vi "main(Test DQMH modules).bak.vi"() -> ()   [LabVIEW 2018, in "Application.lvlib"]
uses:
  eMIC response.ctl
  DRV stand.ctl
  type defs/HW config.ctl
  eMICs Cluster.ctl
  SubVIs/App state data.ctl
  SubVIs/Trigger cluster.ctl
  type defs/DMM all config cluster.ctl
  type defs/DMM config cluster.ctl
  SubVIs/FGV DRV data.ctl
  SubVIs/DUT data Mode.ctl
  Instrument Drivers/LV_driver_MBrelay/type defs/FGV enum.ctl
  SubVIs/Step data.ctl
  DRV cluster 2.ctl
  <vilib>/ErrorRing/Error Ring.xnode
  Application.lvlib
  Switches Module/MB switches Module.lvlib
  MB 01 switches Module/MB 01 switches Module.lvlib
  DMM Module/DMM Module.lvlib
  v2_CE14/CE14_v2.lvlib
  Instrument Drivers/LV_driver_MBrelay/MB Relay.lvlib
panel:
  in  "milliseconds to wait":u32=1500
  in  "Log report":bool
  in  "10-1 delay":u32=70
  in  "6_1 delay2":u32=70
  in  "DMM delay":u32=10
  in  "6_1 delay":u32=150
  in  "1-10delay":u32=70
  in  "eMIC delay":u32=70
  in  "DRV number":u8=1 max=60
  in  "Test Single DRV":bool
  in  "Enum":T1(ring)=enum."Fixxed"
  out "Name":string
  out "SAP ID":string
  out "Progress":string
  out "DRV stand":T2
  in  "Auto/Man":bool
  out "DC Measure Completed":bool caption="DC Completed"
  in  "Test Channel 10":bool
  in  "Test Channel 9":bool
  in  "Test Channel 8":bool
  in  "Test Channel 7":bool
  in  "Test Channel 6":bool
  in  "Test Channel 5":bool
  in  "Test Channel 4":bool
  in  "Test Channel 3":bool
  in  "Test Channel 2":bool
  in  "Test Channel 1":bool
  in  "Shorted Circuits Test":bool
  out "CE14  Module did it":bool[](array[boolean])
  out "time elased(ms)":u32
  out "Inst. 9":bool
  in  "Exit":bool
  out "Inst. 8":bool
  out "Inst. 7":bool
  out "Inst. 6":bool
  out "Inst. 5":bool
  out "Inst. 4":bool
  out "Inst. 3":bool
  out "Inst. 2":bool
  out "Inst. 1":bool
  out "new Trigger?":bool
  out "last Trigger?":bool
  out "error out":errorcluster
  out "State log":string
  out "AC  Completed":bool caption="AC Completed"
  in  "Select CE14 eMIC Module Instance":i32(ring)=-1 items=["All"=-1, "1"=1, "2"=2, "3"=3, "4"=4, "5"=5, "6"=6]
  out "New board?":bool
  in  "Test":bool caption="Again"
  out "DRV 61":u32(colorbox)
  in  "Settings":bool
  in  "VIEW":bool caption="Again"
  out "DRV 60":u32(colorbox) caption="60"
  out "DRV 59":u32(colorbox) caption="59"
  out "DRV 58":u32(colorbox) caption="58"
  out "DRV 57":u32(colorbox) caption="57"
  out "DRV 56":u32(colorbox) caption="56"
  out "DRV 55":u32(colorbox) caption="55"
  out "DRV 54":u32(colorbox) caption="54"
  out "DRV 53":u32(colorbox) caption="53"
  out "DRV 52":u32(colorbox) caption="52"
  out "DRV 51":u32(colorbox) caption="51"
  out "DRV 50":u32(colorbox) caption="50"
  out "DRV 49":u32(colorbox) caption="49"
  out "DRV 48":u32(colorbox) caption="48"
  out "DRV 47":u32(colorbox) caption="47"
  out "DRV 46":u32(colorbox) caption="46"
  out "DRV 45":u32(colorbox) caption="45"
  out "DRV 44":u32(colorbox) caption="44"
  out "DRV 43":u32(colorbox) caption="43"
  out "DRV 42":u32(colorbox) caption="42"
  out "DRV 41":u32(colorbox) caption="41"
  out "DRV 40":u32(colorbox) caption="40"
  out "DRV 39":u32(colorbox) caption="39"
  out "DRV 38":u32(colorbox) caption="38"
  out "DRV 37":u32(colorbox) caption="37"
  out "DRV 36":u32(colorbox) caption="36"
  out "DRV 35":u32(colorbox) caption="35"
  out "DRV 34":u32(colorbox) caption="34"
  out "DRV 33":u32(colorbox) caption="33"
  out "DRV 32":u32(colorbox) caption="32"
  out "DRV 31":u32(colorbox) caption="31"
  out "DRV 30":u32(colorbox) caption="30"
  out "DRV 29":u32(colorbox) caption="29"
  out "DRV 28":u32(colorbox) caption="28"
  out "DRV 27":u32(colorbox) caption="27"
  out "DRV 26":u32(colorbox) caption="26"
  out "DRV 25":u32(colorbox) caption="25"
  out "DRV 24":u32(colorbox) caption="24"
  out "DRV 23":u32(colorbox) caption="23"
  out "DRV 22":u32(colorbox) caption="22"
  out "DRV 21":u32(colorbox) caption="21"
  out "DRV 20":u32(colorbox) caption="20"
  out "DRV 19":u32(colorbox) caption="19"
  out "DRV 18":u32(colorbox) caption="18"
  out "DRV 17":u32(colorbox) caption="17"
  out "DRV 16":u32(colorbox) caption="16"
  out "DRV 15":u32(colorbox) caption="15"
  out "DRV 14":u32(colorbox) caption="14"
  out "DRV 13":u32(colorbox) caption="13"
  out "DRV 12":u32(colorbox) caption="12"
  out "DRV 11":u32(colorbox) caption="11"
  out "DRV 10":u32(colorbox) caption="10"
  out "DRV 9":u32(colorbox) caption="9"
  out "DRV 8":u32(colorbox) caption="8"
  out "DRV 7":u32(colorbox) caption="7"
  out "DRV 6":u32(colorbox) caption="6"
  out "DRV 5":u32(colorbox) caption="5"
  out "DRV 4":u32(colorbox) caption="4"
  out "DRV 3":u32(colorbox) caption="3"
  out "DRV 2":u32(colorbox) caption="2"
  out "DRV 1":u32(colorbox) caption="1"
  out "version":string caption="Version"
  out "Module ID":i32
  in  "Tab Control":T3(tab)
  out "Short DRV":bool[][](array[boolean])
  in  "Mux 10-1":bool
  in  "mux 6-1":bool
  in  "Read Optos":bool
  in  "Select DMM's Current Input":bool
  in  "mux2-1(DMM I) encode":enum16{"DMM I (0.5)", "DMM I (12)"}(ring)
  in  "mux 6-1 data":T4(ring)
  in  "mux 10-1 data":T5(ring)
  in  "set value":bool
  in  "Set trigger value":bool
  out "trigger Value":bool
  in  "Read trigger":bool
  in  "Reset JIG":bool
  in  "eMIC":bool
  in  "DEMUX 1-10":bool
  in  "TurnON/OFF +5V":bool
  in  "5V Value":bool
  in  "demux1_10(x6)_encode":T6(ring)
  in  "eMIC 6 values":bool[](array[boolean])=[FALSE, FALSE, FALSE, FALSE, FALSE, FALSE]
  in  "DMM query":bool
  in  "connect DMM":bool
  in  "DMM read dual value":bool
  in  "config DMM":bool
  in  "Detector Rate":u8(ring)=2 items=["SLOW", "MID", "FAST"]
  in  "DCI range":dbl=0.5
  in  "DCV range":dbl=1000.0
  out "DCV(Volts)":dbl
  out "DCI(mA)":dbl
  out "DMM func?":string
  out "DMM range?":string
  in  "request AC-all":bool
  in  "Open COM eMIC":bool
  in  "check connected":bool
  out "eMIC 1":T7
  out "eMIC 2":T7
  out "eMIC 3":T7
  out "eMIC 4":T7
  out "eMIC 5":T7
  out "eMIC 6":T7
  out "EMIC connected":bool[](array[boolean])
  out "AC switches Module":bool
  out "DC Measure Module":bool
  out "DC Switches Module":bool
  out "AC Measure Module":bool
  # "HV-60D: ON-LINE TESTER FOR LED POWER DRIVER"
  # "60"
  # "6"
  # "12"
  # "18"
  # "24"
  # "30"
  # "36"
  # "42"
  # "48"
  # "54"
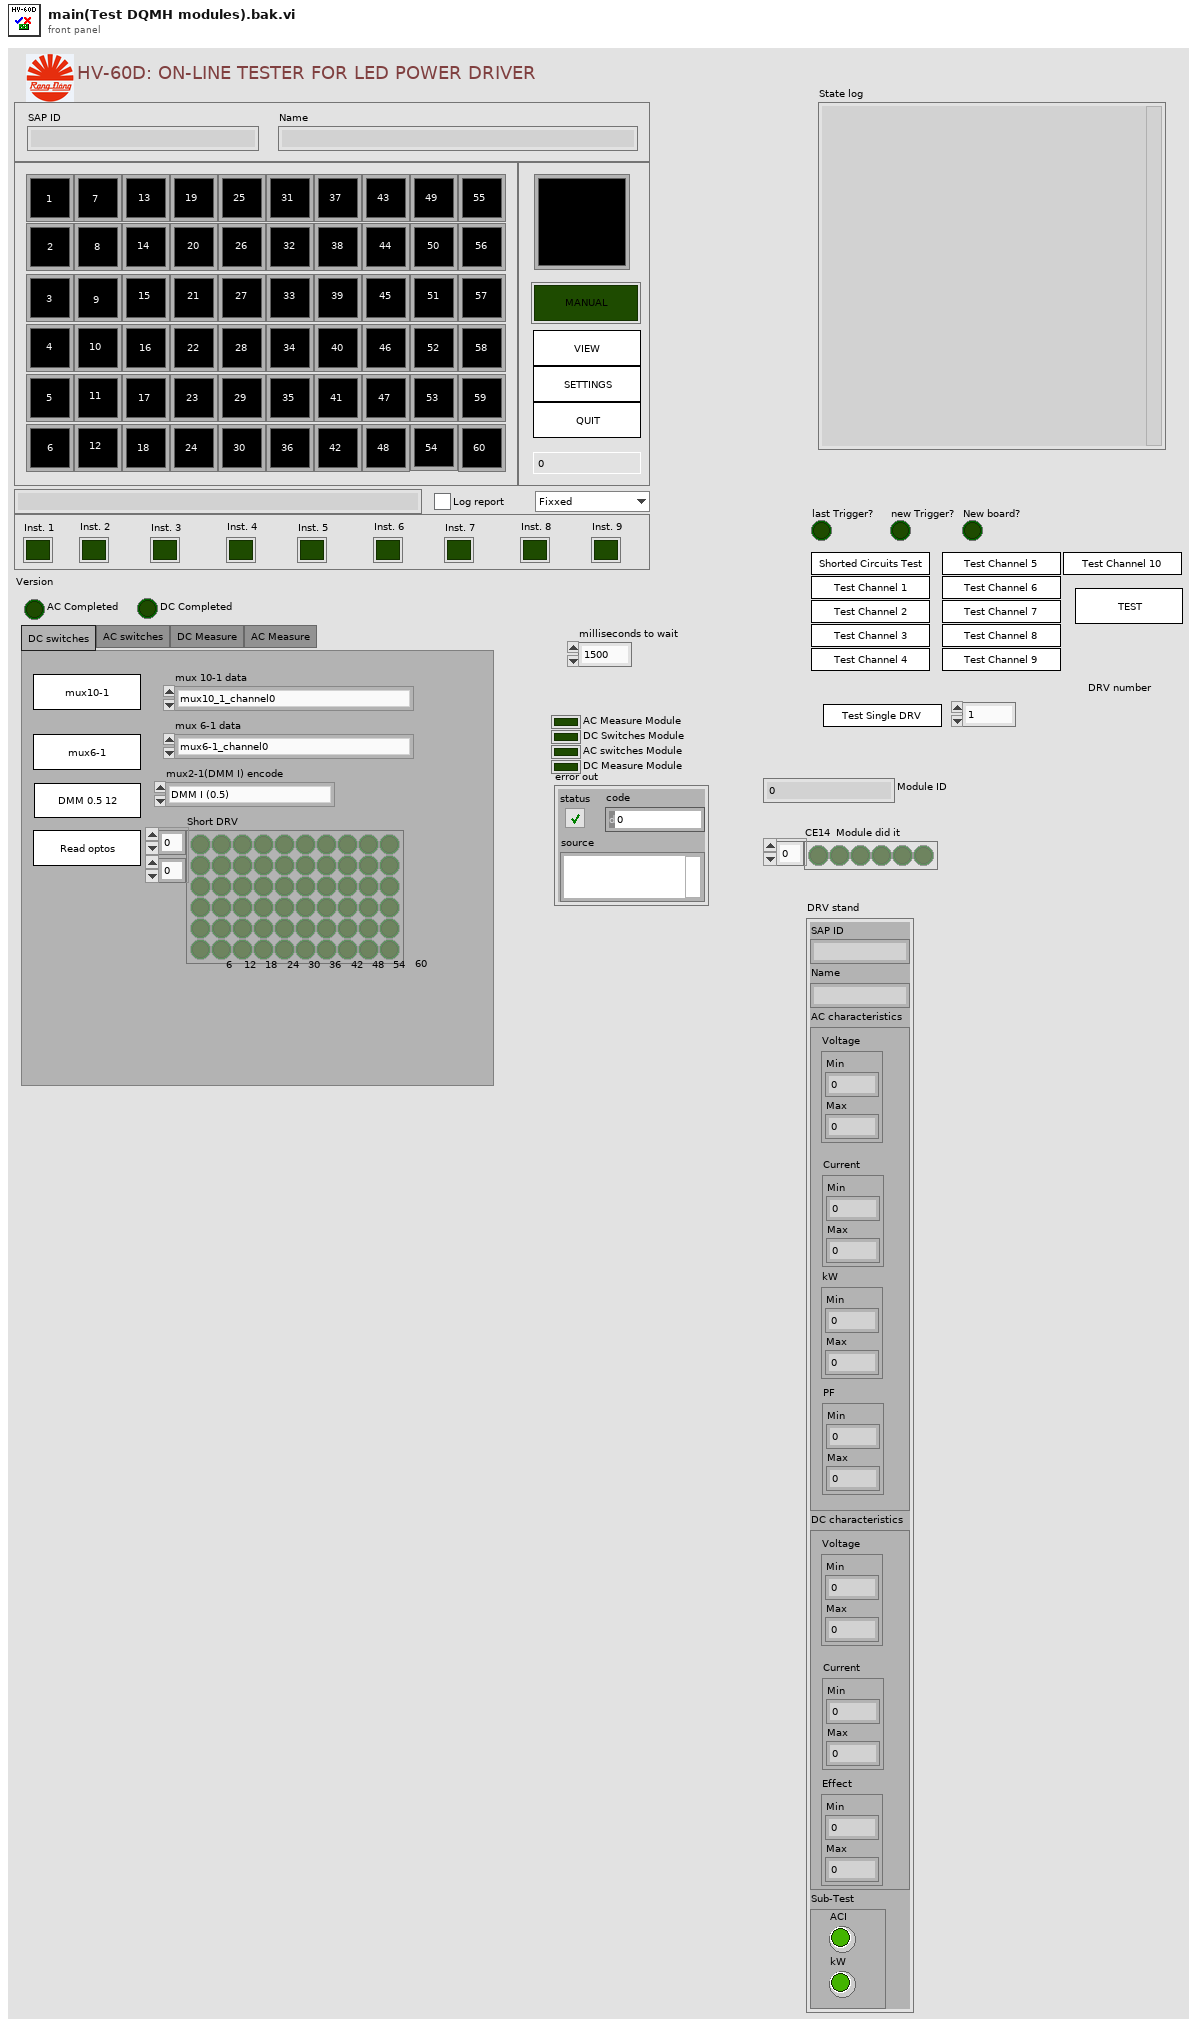
[diagram p1: front panel]
types:
  T1 = enum16{"All DRV", "Fixxed", "Pinpoint_JIG", "00037845(M26)"}
  T2 = typedef "Application.lvlib/DRV stand.ctl" = cluster{"SAP ID":string, "Name":string, "AC characteristics":cluster{"Voltage":cluster{"Min":dbl, "Max":dbl}, "Current":cluster{"Min":dbl, "Max":dbl}, "kW":cluster{"Min":dbl, "Max":dbl}, "PF":cluster{"Min":dbl, "Max":dbl}}, "DC characteristics":cluster{"Voltage":cluster{"Min":dbl, "Max":dbl}, "Current":cluster{"Min":dbl, "Max":dbl}, "Effect":cluster{"Min":dbl, "Max":dbl}}, "Sub-Test":cluster{"ACV":bool, "ACI":bool, "kW":bool, "PF":bool, "DCV":bool, "DCI":bool, "efficiency":bool}}
  T3 = enum32{"DC switches", "AC switches", "DC Measure", "AC Measure"}
  T4 = enum16{"mux6-1_channel0", "mux6_1_channel1_0", "mux6_1_channel1_1", "mux6-1_channel1_2", "mux6_1_channel1_3", "mux6_1_channel2_0", "mux6_1_channel2_1", "mux6_1_channel2_2", "mux6_1_channel2_3", "mux6_1_channel3_0", "mux6_1_channel3_1", "mux6_1_channel3_2", "mux6_1_channel3_3", "mux6_1_channel4_0", "mux6_1_channel4_1", "mux6_1_channel4_2", "mux6_1_channel4_3", "mux6_1_channel5_0", "mux6_1_channel5_1", "mux6_1_channel5_2", "mux6_1_channel5_3", "mux6_1_channel6_0", "mux6_1_channel6_1", "mux6_1_channel6_2", "mux6_1_channel6_3"}
  T5 = enum16{"mux10_1_channel0", "mux10_1_channel1", "mux10_1_channel2", "mux10_1_channel3", "mux10_1_channel4", "mux10_1_channel5", "mux10_1_channel6", "mux10_1_channel7", "mux10_1_channel8", "mux10_1_channel9", "mux10_1_channel10"}
  T6 = enum16{"demux1_10_channel0", "demux1_10_channel1", "demux1_10_channel2", "demux1_10_channel3", "demux1_10_channel4", "demux1_10_channel5", "demux1_10_channel6", "demux1_10_channel7", "demux1_10_channel8", "demux1_10_channel9", "demux1_10_channel10"}
  T7 = typedef "Application.lvlib/eMIC response.ctl" = cluster{"ACV":dbl, "ACI":dbl, "pF":dbl, "kW":dbl, "Freq":dbl, "kvar":dbl}
  T8 = typedef "Application.lvlib/eMICs Cluster.ctl" = cluster{"eMIC 1":T7, "eMIC 2":T7, "eMIC 3":T7, "eMIC 4":T7, "eMIC 5":T7, "eMIC 6":T7}
  T9 = typedef "Application.lvlib/HW config.ctl" = cluster{"DMM":string, "mux":string, "demux":string, "eMIC1":string, "eMIC2":string, "eMIC3":string, "eMIC4":string, "eMIC5":string, "eMIC6":string}
  T10 = typedef "Application.lvlib/Trigger cluster.ctl" = cluster{"new board?":bool, "new trigger":bool, "last trigger":bool}
  T11 = typedef "Application.lvlib/App state data.ctl" = cluster{"command":string, "command data":variant}
  T12 = typedef "CE14_v2.lvlib/Broadcast Events--cluster.ctl" = cluster{"Module Did Init":refnum<user-event>, "Status Updated":refnum<user-event>, "Error Reported":refnum<user-event>, "Module Did Stop":refnum<user-event>, "Update Module Execution Status":refnum<user-event>, "CE14 response data":refnum<user-event>}
  T13 = typedef "MB switches Module.lvlib/Broadcast Events--cluster.ctl" = cluster{"Module Did Init":refnum<user-event>, "Status Updated":refnum<user-event>, "Error Reported":refnum<user-event>, "Module Did Stop":refnum<user-event>, "Update Module Execution Status":refnum<user-event>}
  T14 = typedef "MB 01 switches Module.lvlib/Broadcast Events--cluster.ctl" = cluster{"Module Did Init":refnum<user-event>, "Status Updated":refnum<user-event>, "Error Reported":refnum<user-event>, "Module Did Stop":refnum<user-event>, "Update Module Execution Status":refnum<user-event>}
  T15 = typedef "DMM Module.lvlib/Broadcast Events--cluster.ctl" = cluster{"Module Did Init":refnum<user-event>, "Status Updated":refnum<user-event>, "Error Reported":refnum<user-event>, "Module Did Stop":refnum<user-event>, "Update Module Execution Status":refnum<user-event>}
  T16 = enum16{"open", "replace", "create", "open or create", "replace or create", "replace or create with confirmation"}
  T17 = typedef "Application.lvlib/DRV cluster 2.ctl" = cluster{"Shorted Circuit":bool, "AC voltage(volts)":dbl, "AC Current (mA)":dbl, "AC kW (W)":dbl, "AC pF ":dbl, "DC Voltage (Volts)":dbl, "DC Current (mA)":dbl, "DC kW (W)":dbl, "DRV Fail/Pass (T)":bool, "efficient (%)":dbl}
  T18 = enum32{"Invalid", "Standard", "Closed", "Hidden", "Minimized", "Maximized"}
  T19 = typedef "Application.lvlib/DMM all config cluster.ctl" = cluster{"DMM config cluster":T20, "mux2-1(DMM I) encode":enum16{"DMM I (0.5)", "DMM I (12)"}}
  T20 = typedef "Application.lvlib/DMM config cluster.ctl" = cluster{"DCV range":dbl, "DCI range":dbl, "Detector Rate":u8}
  T21 = typedef "Application.lvlib/DUT data Mode.ctl" = enum16{"range Limit", "Short Circuits", "AC parameter", "AC parameter 1", "DC parameter"}
  T22 = typedef "Application.lvlib/FGV DRV data.ctl" = enum16{"Init", "Write", "Read", "Process"}
  T23 = typedef "MB Relay.lvlib/FGV enum.ctl" = enum16{"Write", "Init FGV", "Read", "All OFF", "All ON"}
  T24 = typedef "CE14_eMIC.lvlib/CE14.data.ctl" = cluster{"string":string, "float":dbl, "Name":string}
  T25 = typedef "Application.lvlib/Step data.ctl" = cluster{"command":string, "Data":variant}
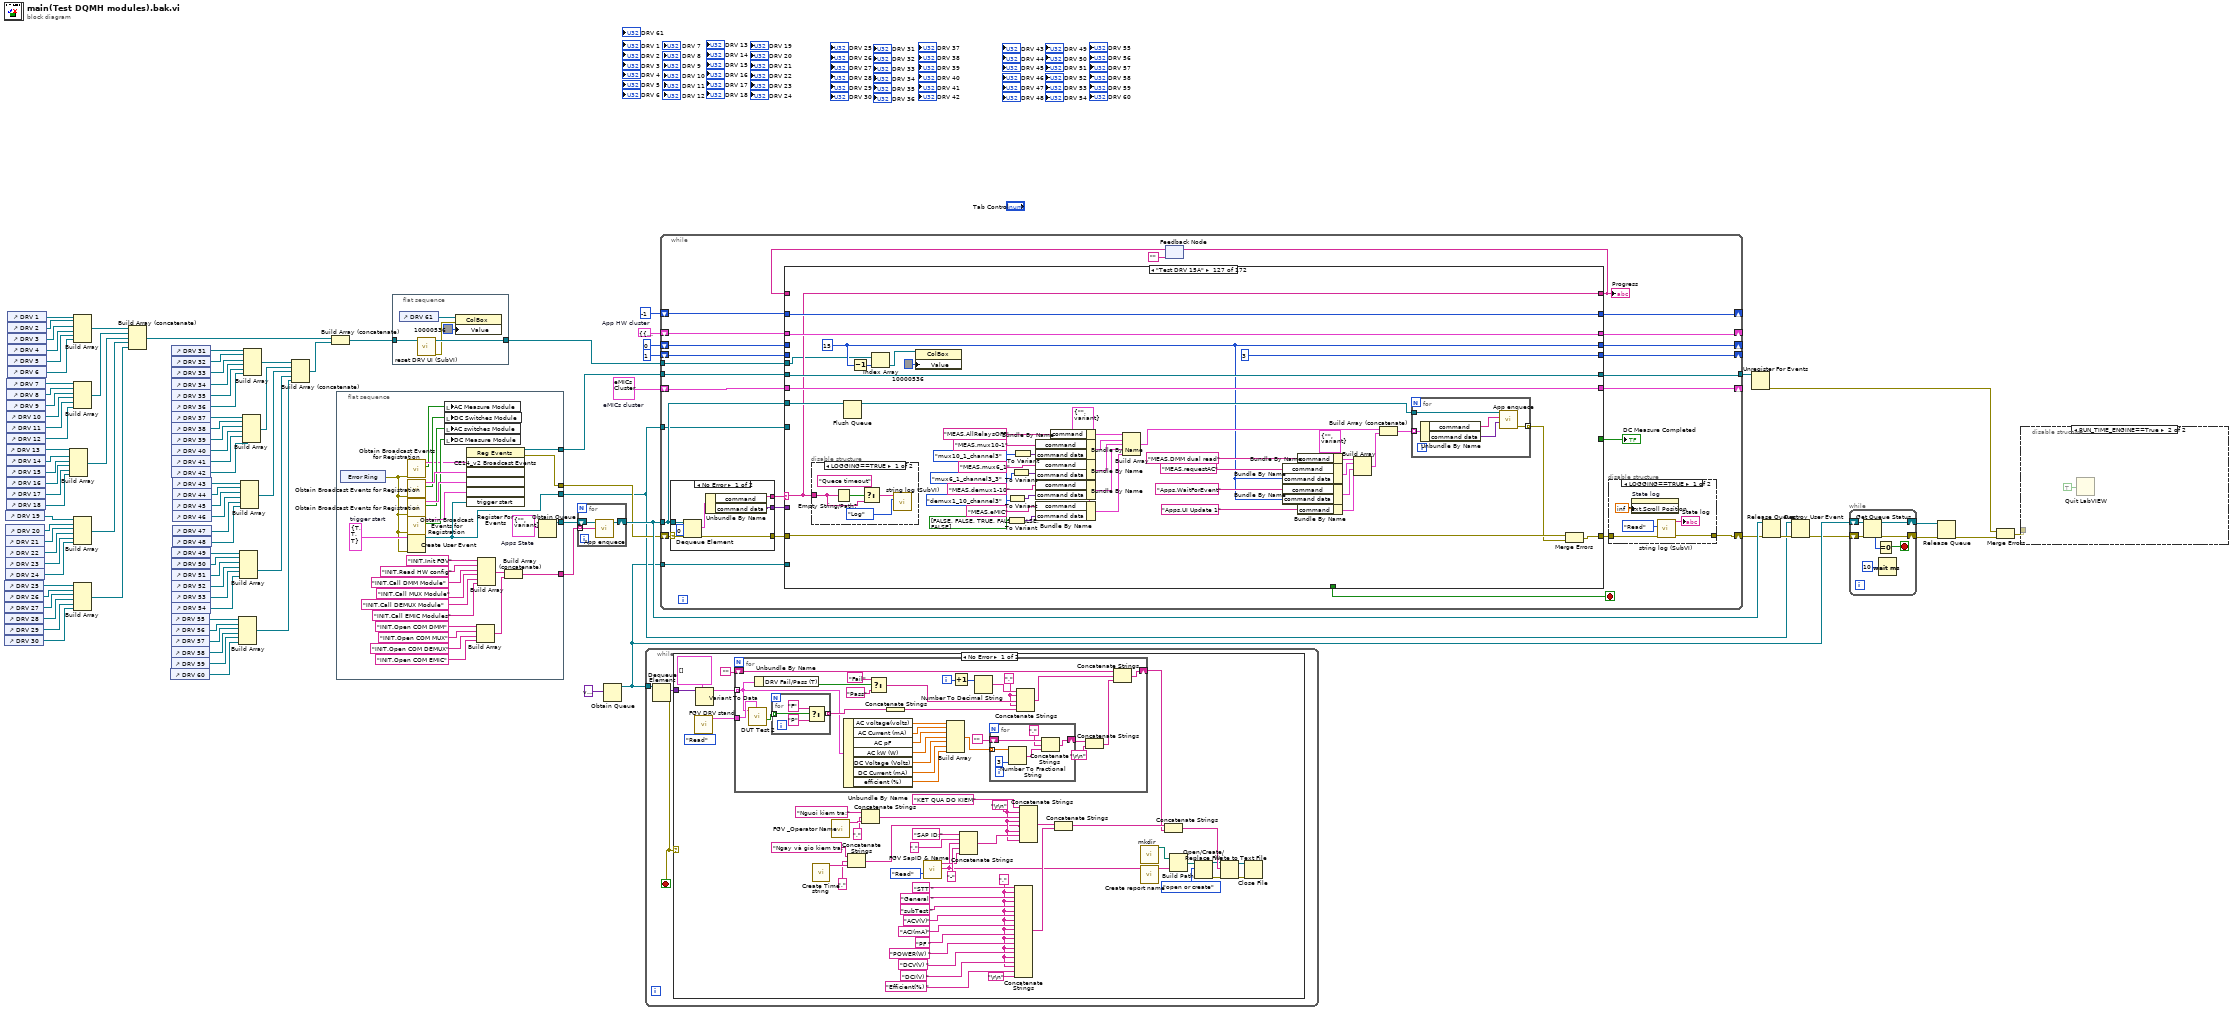
[diagram p0: block diagram]
diagram:
  w88 = T8 {"eMIC 1"={"ACV"=0.0, "ACI"=0.0, "pF"=0.0, "kW"=0.0, "Freq"=0.0, "kvar"=0.0}, "eMIC 2"={"ACV"=0.0, "ACI"=0.0, "pF"=0.0, "kW"=0.0, "Freq"=0.0, "kvar"=0.0}, "eMIC 3"={"ACV"=0.0, "ACI"=0.0, "pF"=0.0, "kW"=0.0, "Freq"=0.0, "kvar"=0.0}, "eMIC 4"={"ACV"=0.0, "ACI"=0.0, "pF"=0.0, "kW"=0.0, "Freq"=0.0, "kvar"=0.0}, "eMIC 5"={"ACV"=0.0, "ACI"=0.0, "pF"=0.0, "kW"=0.0, "Freq"=0.0, "kvar"=0.0}, "eMIC 6"={"ACV"=0.0, "ACI"=0.0, "pF"=0.0, "kW"=0.0, "Freq"=0.0, "kvar"=0.0}}  # eMICs cluster
  w93 = cluster{"HW config 2":T9} {"HW config 2"={"DMM"="COM15", "mux"="COM11", "demux"="COM16", "eMIC1"="COM13", "eMIC2"="COM6", "eMIC3"="COM9", "eMIC4"="COM10", "eMIC5"="COM12", "eMIC6"="COM11"}}  # App HW cluster
  n1 = control-ref of="DRV 25"() -> (w58:refnum<vi>)
  n2 = control-ref of="DRV 26"() -> (w59:refnum<vi>)
  n3 = control-ref of="DRV 27"() -> (w60:refnum<vi>)
  n4 = control-ref of="DRV 28"() -> (w61:refnum<vi>)
  n5 = control-ref of="DRV 29"() -> (w62:refnum<vi>)
  n6 = control-ref of="DRV 30"() -> (w63:refnum<vi>)
  n7 = control-ref of="DRV 21"() -> (w67:refnum<vi>)
  n8 = control-ref of="DRV 22"() -> (w66:refnum<vi>)
  n9 = control-ref of="DRV 23"() -> (w65:refnum<vi>)
  n10 = control-ref of="DRV 24"() -> (w64:refnum<vi>)
  n11 = control-ref of="DRV 19"() -> (w69:refnum<vi>)
  n12 = control-ref of="DRV 20"() -> (w68:refnum<vi>)
  n13 = control-ref of="DRV 13"() -> (w75:refnum<vi>)
  n14 = control-ref of="DRV 7"() -> (w81:refnum<vi>)
  n15 = control-ref of="DRV 8"() -> (w80:refnum<vi>)
  n16 = control-ref of="DRV 9"() -> (w79:refnum<vi>)
  n17 = control-ref of="DRV 10"() -> (w78:refnum<vi>)
  n18 = control-ref of="DRV 11"() -> (w77:refnum<vi>)
  n19 = control-ref of="DRV 12"() -> (w76:refnum<vi>)
  n20 = control-ref of="DRV 14"() -> (w74:refnum<vi>)
  n21 = control-ref of="DRV 15"() -> (w73:refnum<vi>)
  n22 = control-ref of="DRV 16"() -> (w72:refnum<vi>)
  n23 = control-ref of="DRV 17"() -> (w71:refnum<vi>)
  n24 = control-ref of="DRV 18"() -> (w70:refnum<vi>)
  n25 = control-ref of="DRV 1"() -> (w87:refnum<vi>)
  n26 = control-ref of="DRV 2"() -> (w86:refnum<vi>)
  n27 = control-ref of="DRV 3"() -> (w85:refnum<vi>)
  n28 = control-ref of="DRV 4"() -> (w84:refnum<vi>)
  n29 = control-ref of="DRV 5"() -> (w83:refnum<vi>)
  n30 = control-ref of="DRV 6"() -> (w82:refnum<vi>)
  n31 = Build Array(w75, w74, w73, w72, w71, w70) -> (w55:refnum<vi>[])
  n32 = Build Array(w87, w86, w85, w84, w83, w82) -> (w57:refnum<vi>[])
  n33 = Build Array(w69, w68, w67, w66, w65, w64) -> (w54:refnum<vi>[])
  n34 = Build Array(w58, w59, w60, w61, w62, w63) -> (w53:refnum<vi>[])
  n35 = Build Array(w81, w80, w79, w78, w77, w76) -> (w56:refnum<vi>[])
  n36 = Build Array (concatenate)(w57, w56, w55, w54, w53) -> (w17:refnum<vi>[])
  n37 = control-ref of="DRV 60"() -> (w28:refnum<vi>)
  n38 = control-ref of="DRV 55"() -> (w23:refnum<vi>)
  n39 = control-ref of="DRV 56"() -> (w24:refnum<vi>)
  n40 = control-ref of="DRV 57"() -> (w25:refnum<vi>)
  n41 = control-ref of="DRV 58"() -> (w26:refnum<vi>)
  n42 = control-ref of="DRV 59"() -> (w27:refnum<vi>)
  n43 = control-ref of="DRV 31"() -> (w47:refnum<vi>)
  n44 = control-ref of="DRV 32"() -> (w48:refnum<vi>)
  n45 = control-ref of="DRV 33"() -> (w49:refnum<vi>)
  n46 = control-ref of="DRV 34"() -> (w50:refnum<vi>)
  n47 = control-ref of="DRV 35"() -> (w51:refnum<vi>)
  n48 = control-ref of="DRV 36"() -> (w52:refnum<vi>)
  n49 = control-ref of="DRV 37"() -> (w46:refnum<vi>)
  n50 = control-ref of="DRV 38"() -> (w45:refnum<vi>)
  n51 = control-ref of="DRV 39"() -> (w44:refnum<vi>)
  n52 = control-ref of="DRV 40"() -> (w43:refnum<vi>)
  n53 = control-ref of="DRV 41"() -> (w42:refnum<vi>)
  n54 = control-ref of="DRV 42"() -> (w41:refnum<vi>)
  n55 = control-ref of="DRV 49"() -> (w34:refnum<vi>)
  n56 = control-ref of="DRV 50"() -> (w33:refnum<vi>)
  n57 = control-ref of="DRV 51"() -> (w32:refnum<vi>)
  n58 = control-ref of="DRV 52"() -> (w31:refnum<vi>)
  n59 = control-ref of="DRV 53"() -> (w30:refnum<vi>)
  n60 = control-ref of="DRV 54"() -> (w29:refnum<vi>)
  n61 = control-ref of="DRV 43"() -> (w35:refnum<vi>)
  n62 = control-ref of="DRV 44"() -> (w36:refnum<vi>)
  n63 = control-ref of="DRV 45"() -> (w37:refnum<vi>)
  n64 = control-ref of="DRV 46"() -> (w38:refnum<vi>)
  n65 = control-ref of="DRV 47"() -> (w39:refnum<vi>)
  n66 = control-ref of="DRV 48"() -> (w40:refnum<vi>)
  n67 = Build Array(w23, w24, w25, w26, w27, w28) -> (w18:refnum<vi>[])
  n68 = Build Array(w34, w33, w32, w31, w30, w29) -> (w19:refnum<vi>[])
  n69 = Build Array(w35, w36, w37, w38, w39, w40) -> (w20:refnum<vi>[])
  n70 = Build Array(w46, w45, w44, w43, w42, w41) -> (w21:refnum<vi>[])
  n71 = Build Array(w47, w48, w49, w50, w51, w52) -> (w22:refnum<vi>[])
  n72 = Build Array (concatenate)(w22, w21, w20, w19, w18) -> (w16:refnum<vi>[])
  n73 = Build Array (concatenate)(w17, w16) -> (w14:refnum<vi>[])
  n74 = flat-sequence {
    tunnel: [w118] -> w95
    tunnel: [w117] -> w92
    tunnel: [w116] -> w91
    tunnel: [w115] -> w15
    tunnel: [w110] -> w7
    frame #0 {
      w111 = T10 {"new board?"=TRUE, "new trigger"=TRUE, "last trigger"=TRUE}  # trigger start
      w112 = T11 {"command"="", "command data"=variant}  # Apps State
      n75 = xnode "Error Ring"() -> ("error out"=w109:errorcluster)
      n76 = call "Obtain Broadcast Events for Registration.vi"("error in (no error)"=w109) -> ("Already running?"=w113:bool, "CE14_v2 Broadcast Events"=w114:T12)  [unwired: 8 in, 1 out]
      n77 = call "Obtain Broadcast Events for Registration.vi"("error in (no error)"=w109) -> ("Already running?"=w121:bool, "Switches Module Broadcast Events"=w124:T13)  [unwired: 8 in, 1 out]
      n78 = call "Obtain Broadcast Events for Registration.vi"("error in (no error)"=w109) -> ("Already running?"=w120:bool, "MB 01 switches Module Broadcast Events"=w123:T14)  [unwired: 8 in, 1 out]
      n79 = call "Obtain Broadcast Events for Registration.vi"("error in (no error)"=w109) -> ("Already running?"=w119:bool, "DMM Module Broadcast Events"=w122:T15)  [unwired: 8 in, 1 out]
      n80 = Create User Event(user event datatype=w111, error in=w109) -> (user event=w110:refnum<user-event>)  [unwired: 1 out]
      n81 = local write "AC Measure Module"(w113) -> ()
      n82 = local write "DC Switches Module"(w121) -> ()
      n83 = local write "AC switches Module"(w120) -> ()
      n84 = local write "DC Measure Module"(w119) -> ()
      n85 = register-events(w114, w124, w123, w122, w110) -> (reference out=w118:refnum<event-registration>, error out=w115:errorcluster)  [unwired: 2 in]
      n86 = Build Array("INIT.Open COM DMM", "INIT.Open COM MUX", "INIT.Open COM DEMUX", "INIT.Open COM EMIC") -> (w106:string[])
      n87 = Build Array("INIT.Init FGV", "INIT.Read HW config", "INIT.Call DMM Module", "INIT.Call MUX Module", "INIT.Call DEMUX Module", "INIT.Call EMIC Modules") -> (w107:string[])
      n88 = Build Array (concatenate)(w107, w106) -> (w116:string[])
      n89 = Obtain Queue(element data type=w112) -> (queue out=w117:refnum<queue>)  [unwired: 4 in, 2 out]
    }
  }
  n90 = flat-sequence {
    tunnel: w14 -> [w130]
    tunnel: [w129] -> w13
    frame #0 {
      n91 = control-ref of="DRV 61"() -> (w126:refnum<vi>)
      n92 = call "reset DRV UI (SubVI).vi"("Ref  in"=w130) -> ("error out"=w127:errorcluster, "Ref out"=w129:refnum<vi>[])  [unwired: 9 in]
      n93 = property class="ColBox"(reference=w126, error in=w127, "Value"=u32 10000536 ("DRV 1")) -> ()  [unwired: 2 out]
    }
  }
  n94 = for {
    tunnel: w91 -> [w133] mode=indexing
    shift-right: [w131] -> w90
    shift-left: w92 -> [w132]
    n95 = call "App enquece.vi"("command"=w133, "queue in"=w132) -> ("Queue out"=w131:refnum<queue>)  [unwired: 8 in, 1 out]
  }
  n96 = Obtain Queue(element data type=variant) -> (queue out=w5:refnum<queue>)  [unwired: 4 in, 2 out]
  n97 = while {
    tunnel: w5 -> [w136]
    stop <- w134 stop-if-true
    n98 = Dequeue Element(queue=w136) -> (element=w135:variant, error out=w134:errorcluster)  [unwired: 2 in, 2 out]
    n99 = case shown="No Error" w134 {
      tunnel: w135 -> [w183 _]
      frame No Error {
        w148 = ","
        w156 = "\r\n"
        n100 = call "FGV DRV stand.vi"("Enum"=enum16{"Write", "Read"}."Read" ("Enum 2")) -> ("DRV stand out"=w180:T2)  [unwired: 10 in]
        n101 = Variant To Data(type=T17[] [] ("60 DRV data"), Variant=w183) -> (data=w182:T17[])  [unwired: 1 in, 1 out]
        n102 = for {
          tunnel: w182 -> [w201] mode=indexing
          tunnel: w180 -> [w212]
          shift-right: [w189] -> w158
          shift-left: "" -> [w188]
          i -> [w206]
          w185 = ","
          n103 = call "DUT Test 2.vi"("DRV stand"=w212, "DRV data"=w201) -> ("actual subtest"=w208:bool[])  [unwired: 6 in, 3 out]
          n104 = Unbundle By Name(w201) -> ("DRV Fail/Pass (T)"=w211:bool)
          n105 = for {
            tunnel: w208 -> [w221] mode=indexing
            tunnel: [w220] -> w207 mode=indexing
            n106 = Select(t="F", s=w221, f="P") -> (s? t:f=w220:string)
          }
          n107 = Unbundle By Name(w201) -> ("AC voltage(volts)"=w200:dbl, "AC Current (mA)"=w199:dbl, "AC pF"=w198:dbl, "AC kW (W)"=w197:dbl, "DC Voltage (Volts)"=w196:dbl, "DC Current (mA)"=w195:dbl, "efficient (%)"=w194:dbl)
          n108 = Select(t="Fail", s=w211, f="Pass") -> (s? t:f=w203:string)
          n109 = Concatenate Strings(w207) -> (w202:string)
          n110 = Build Array(w200, w199, w198, w197, w196, w195, w194) -> (w193:dbl[])
          n111 = Increment(x=w206) -> (x+1=w205:i32)
          n112 = Number To Decimal String(number=w205) -> (decimal integer string=w204:string)  [unwired: 1 in]
          n113 = for {
            tunnel: w193 -> [w218] mode=indexing
            shift-right: [w215] -> w191
            shift-left: "" -> [w216]
            n114 = Number To Fractional String(number=w218, precision (6)=i16 3) -> (F-format string=w214:string)  [unwired: 2 in]
            n115 = Concatenate Strings(w216, ",", w214) -> (w215:string)
          }
          n116 = Concatenate Strings(w204, w185, w203, w185, w202) -> (w187:string)
          n117 = Concatenate Strings(w191, "\r\n") -> (w186:string)
          n118 = Concatenate Strings(w188, w187, w186) -> (w189:string)
        }
        n119 = call "Create Time string.vi"() -> ("Timestr"=w154:string)  [unwired: 10 in, 1 out]
        n120 = call "FGV _Operator Name.vi"() -> ("Operator Name out"=w178:string)  [unwired: 11 in]
        n121 = Concatenate Strings("Ngay và gio kiem tra:", ",", w154) -> (w153:string)
        n122 = Concatenate Strings("Nguoi kiem tra:", ",", w178) -> (w179:string)
        n123 = call "FGV SapID & Name.vi"("Enum"=enum16{"Read", "Write"}."Read") -> ("SAP ID 2"=w137:string, "Name 2"=w138:string)  [unwired: 8 in, 1 out]
        n124 = Concatenate Strings("SAP ID:", ",", w137, "-", w138) -> (w157:string)
        n125 = Concatenate Strings("STT ", w148, "General ", w148, "subTest ", w148, "ACV(V)", w148, "ACI(mA)", w148, "PF ", w148, "POWER(W) ", w148, "DCV(V) ", w148, "DCI(V) ", w148, "Efficient(%) ", "\r\n") -> (w161:string)
        n126 = Concatenate Strings("KET QUA DO KIEM" ("string"), w156, w179, w156, w153, w156, w157, w156) -> (w160:string)
        n127 = Concatenate Strings(w160, w161) -> (w159:string)
        n128 = call "mkdir.vi"() -> ("created path"=w147:path)  [unwired: 10 in, 1 out]
        n129 = call "Create report name.vi"("SAP ID"=w137) -> ("filename"=w146:string)  [unwired: 9 in, 1 out]
        n130 = Concatenate Strings(w159, w158) -> (w143:string)
        n131 = Build Path(base path=w147, name or relative path=w146) -> (appended path=w145:path)
        n132 = Open/Create/Replace File(file path (use dialog)=w145, operation (0:open)=T16."open or create") -> (refnum out=w142:refnum<file>, error out=w141:errorcluster)  [unwired: 4 in, 1 out]
        n133 = Write to Text File(file (use dialog)=w142, text=w143, error in=w141) -> (refnum out=w139:refnum<file>, error out=w140:errorcluster)  [unwired: 1 in, 1 out]
        n134 = Close File(refnum=w139, error in=w140) -> ()  [unwired: 2 out]
      }
      frame Error {
      }
    }
  }
  n135 = while {
    shift-right: [w227] -> w89
    shift-left: w15 -> [w249]
    shift-right: [w247] -> _
    shift-left: -1 -> [w246]
    tunnel: w95 -> [w245]
    tunnel: [w244] -> w94
    shift-right: [w242] -> _
    shift-left: w93 -> [w243]
    tunnel: w90 -> [w231]
    shift-right: [w240] -> _
    shift-left: w88 -> [w239]
    tunnel: w13 -> [w237]
    shift-right: [w236] -> _
    shift-left: 1 ("DUT channel (1-11)") -> [w235]
    shift-right: [w234] -> _
    shift-left: 0 ("DUT index(0-59)") -> [w233]
    tunnel: w7 -> [w230]
    tunnel: w5 -> [w223]
    stop <- w238 stop-if-true
    n136 = case shown="No Error" w249 {
      selector: w249 -> [w261 w262]
      tunnel: [w259 "Apps.Error Handler"] -> w232
      tunnel: [w260 w262] -> w248
      tunnel: [w258 _] -> w241
      tunnel: w231 -> [w257 _]
      frame No Error {
        n137 = Dequeue Element(queue=w257, timeout in ms (-1)=0, error in (no error)=w261) -> (element=w256:T11, error out=w260:errorcluster)  [unwired: 2 out]
        n138 = Unbundle By Name(w256) -> ("command"=w259:string, "command data"=w258:variant)
      }
      frame Error {
      }
    }
    n139 = feedback #1("") -> (w225:string)
    n140 = case shown="\"Test DRV 15A\"" w232 {
      selector: w232 -> [w272 _ _ w1329 w1349 w1415 w1440 w1494 _ _ _ w1572 w1595 _ w1646 w1719 w1734 w1757 w1780 w1805 w1839 w1858 w1877 w1896 w1929 w1959 w1984 w2013 w2046 w2067 w2091 w2126 w2142 w2167 w2202 w2235 w2274 w2324 w2364 w2409 w2464 w2536 w2606 w2677 w2748 w2819 w2890 w2961 w3033 w3106 w3183 w3233 w3272 w3313 w3354 w3395 w3434 w3477 w3518 w3559 w3600 w3641 w3682 w3723 w3764 w3805 w3846 w3887 w3926 w3969 w4010 w4051 w4092 w4133 w4174 w4215 w4256 w4297 w4338 w4379 w4420 w4461 w4502 w4543 w4584 w4625 w4666 w4707 w4748 w4789 w4830 w4871 w4912 w4953 w4994 w5035 w5076 w5117 w5158 w5199 w5240 w5281 w5322 w5363 w5404 w5445 w5486 w5527 w5568 w5609 w5650 _ w5707 w5764 w5821 w5878 w5935 w5992 w6049 w6106 w6163 w6220 w6277 w6334 w6391 w6448 w6506 w6563 w6620 w6677 w6734 w6791 w6848 w6905 w6962 w7019 w7076 w7133 w7190 w7247 w7304 w7361 w7418 w7475 w7532 w7589 w7646 w7703 w7760 w7818 w7874 w7931 w7988 w8045 w8102 w8159 w8216 w8273 w8332 w8387 w8444 w8501 w8558 w8615 w8673 w8729 w8786 w8843 w8903 w8962 w9021 w9080]
      tunnel: w248 -> [w278 w1314 w1317 w1330 w1356 w1417 w1453 w1502 w1546 w1549 w1570 w1580 w1609 w1639 w1658 w1720 w1735 w1758 w1781 w1806 w1840 w1859 w1878 w1897 w1932 w1960 w1985 w2014 w2049 w2070 w2090 w2127 w2143 w2168 w2203 w2240 w2277 w2327 w2365 w2403 w2466 w2538 w2608 w2679 w2750 w2821 w2892 w2963 w3035 w3108 w3185 w3236 w3277 w3318 w3359 w3400 w3441 w3482 w3523 w3564 w3605 w3646 w3687 w3728 w3769 w3810 w3851 w3892 w3933 w3974 w4015 w4056 w4097 w4138 w4179 w4220 w4261 w4302 w4343 w4384 w4425 w4466 w4507 w4548 w4589 w4630 w4671 w4712 w4753 w4794 w4835 w4876 w4917 w4958 w4999 w5040 w5081 w5122 w5163 w5204 w5245 w5286 w5327 w5368 w5409 w5450 w5491 w5532 w5573 w5614 w5655 w5696 w5713 w5770 w5827 w5884 w5941 w5998 w6055 w6112 w6169 w6226 w6283 w6340 w6397 w6454 w6512 w6569 w6626 w6683 w6740 w6797 w6854 w6911 w6968 w7025 w7082 w7139 w7196 w7253 w7310 w7367 w7424 w7481 w7538 w7595 w7652 w7709 w7766 w7823 w7880 w7937 w7994 w8051 w8108 w8165 w8222 w8279 w8324 w8393 w8450 w8507 w8564 w8621 w8679 w8735 w8792 w8849 w8909 w8968 w9027 w9086]
      tunnel: [w279 w1314 w1318 w1331 w1357 w1418 w1433 w1493 w1546 w1548 w1570 w1581 w1597 w1628 w1649 w1710 w1736 w1759 w1782 w1804 w1838 w1857 w1876 w1895 w1921 w1958 w1982 w2010 w2048 w2069 w2093 w2122 w2147 w2170 w2206 w2238 w2276 w2325 w2363 w2397 w2467 w2539 w2609 w2680 w2751 w2822 w2893 w2964 w3036 w3109 w3186 w3237 w3278 w3319 w3360 w3401 w3442 w3483 w3524 w3565 w3606 w3647 w3688 w3729 w3770 w3811 w3852 w3893 w3934 w3975 w4016 w4057 w4098 w4139 w4180 w4221 w4262 w4303 w4344 w4385 w4426 w4467 w4508 w4549 w4590 w4631 w4672 w4713 w4754 w4795 w4836 w4877 w4918 w4959 w5000 w5041 w5082 w5123 w5164 w5205 w5246 w5287 w5328 w5369 w5410 w5451 w5492 w5533 w5574 w5615 w5656 w5696 w5711 w5768 w5825 w5882 w5939 w5996 w6053 w6110 w6167 w6224 w6281 w6338 w6395 w6452 w6510 w6567 w6624 w6681 w6738 w6795 w6852 w6909 w6966 w7023 w7080 w7137 w7194 w7251 w7308 w7365 w7422 w7479 w7536 w7593 w7650 w7707 w7764 w7821 w7878 w7935 w7992 w8049 w8106 w8163 w8220 w8277 w8335 w8391 w8448 w8505 w8562 w8619 w8677 w8733 w8790 w8847 w8907 w8966 w9025 w9084] -> w228
      tunnel: [_ _ _ _ _ _ _ _ _ _ _ TRUE _ _ _ _ _ _ _ _ _ _ _ _ _ _ _ _ _ _ _ _ _ _ _ _ _ _ _ _ _ _ _ _ _ _ _ _ _ _ _ _ _ _ _ _ _ _ _ _ _ _ _ _ _ _ _ _ _ _ _ _ _ _ _ _ _ _ _ _ _ _ _ _ _ _ _ _ _ _ _ _ _ _ _ _ _ _ _ _ _ _ _ _ _ _ _ _ _ _ _ _ _ _ _ _ _ _ _ _ _ _ _ _ _ _ _ _ _ _ _ _ _ _ _ _ _ _ _ _ _ _ _ _ _ _ _ _ _ _ _ _ _ _ _ _ _ _ _ _ _ _ _ _ _ _ _ _ _ _ _ _] -> w238
      tunnel: [w283 100 w1327 w1340 w1360 w1421 w1434 w1501 w1545 w1557 w1569 w1587 w1608 w1638 w1657 w1727 w1750 w1773 w1796 w1820 w1847 w1866 w1885 w1905 w1938 w1974 w1993 w2020 w2037 w2080 w2099 w2123 w2154 w2178 w2221 w2246 w2285 w2335 w2370 w2427 w2486 w2557 w2628 w2699 w2770 w2841 w2912 w2983 w3054 w3125 w3202 w3242 w3283 w3324 w3365 w3406 w3447 w3488 w3529 w3570 w3611 w3652 w3693 w3734 w3775 w3816 w3857 w3898 w3939 w3980 w4021 w4062 w4103 w4144 w4185 w4226 w4267 w4308 w4349 w4390 w4431 w4472 w4513 w4554 w4595 w4636 w4677 w4718 w4759 w4800 w4841 w4882 w4923 w4964 w5005 w5046 w5087 w5128 w5169 w5210 w5251 w5292 w5333 w5374 w5415 w5456 w5497 w5538 w5579 w5620 w5661 w5695 w5743 w5800 w5857 w5914 w5971 w6028 w6085 w6142 w6199 w6256 w6313 w6370 w6427 w6484 w6541 w6598 w6655 w6712 w6769 w6826 w6883 w6940 w6997 w7054 w7111 w7168 w7225 w7282 w7339 w7396 w7453 w7510 w7567 w7624 w7681 w7738 w7795 w7852 w7909 w7966 w8023 w8080 w8137 w8194 w8251 w8308 w8365 w8422 w8479 w8536 w8593 w8650 w8707 w8764 w8821 w8878 w8937 w8996 w9055 w9114] -> w247
      tunnel: w246 -> [w271 _ w1327 w1340 w1360 w1421 w1434 w1501 w1545 w1557 w1569 w1587 w1608 w1638 w1657 w1727 w1750 w1773 w1796 w1820 w1847 w1866 w1885 w1905 w1938 w1974 w1993 w2020 w2036 w2080 w2099 w2123 w2154 w2178 w2221 w2246 w2285 w2335 w2370 w2427 w2486 w2557 w2628 w2699 w2770 w2841 w2912 w2983 w3054 w3125 w3202 w3242 w3283 w3324 w3365 w3406 w3447 w3488 w3529 w3570 w3611 w3652 w3693 w3734 w3775 w3816 w3857 w3898 w3939 w3980 w4021 w4062 w4103 w4144 w4185 w4226 w4267 w4308 w4349 w4390 w4431 w4472 w4513 w4554 w4595 w4636 w4677 w4718 w4759 w4800 w4841 w4882 w4923 w4964 w5005 w5046 w5087 w5128 w5169 w5210 w5251 w5292 w5333 w5374 w5415 w5456 w5497 w5538 w5579 w5620 w5661 w5695 w5743 w5800 w5857 w5914 w5971 w6028 w6085 w6142 w6199 w6256 w6313 w6370 w6427 w6484 w6541 w6598 w6655 w6712 w6769 w6826 w6883 w6940 w6997 w7054 w7111 w7168 w7225 w7282 w7339 w7396 w7453 w7510 w7567 w7624 w7681 w7738 w7795 w7852 w7909 w7966 w8023 w8080 w8137 w8194 w8251 w8308 w8365 w8422 w8479 w8536 w8593 w8650 w8707 w8764 w8821 w8878 w8937 w8996 w9055 w9114]
      tunnel: w245 -> [w282 w1313 w1326 w1339 w1359 w1420 w1452 w1500 w1544 w1556 w1568 w1586 w1607 w1637 w1656 w1726 w1748 w1771 w1794 w1813 w1846 w1865 w1884 w1904 w1937 w1973 w1992 w2019 w2055 w2079 w2098 w2133 w2153 w2177 w2220 w2245 w2284 w2334 w2369 w2426 w2485 w2556 w2627 w2698 w2769 w2840 w2911 w2982 w3016 w3124 w3201 w3241 w3282 w3323 w3364 w3405 w3446 w3487 w3528 w3569 w3610 w3651 w3692 w3733 w3774 w3815 w3856 w3897 w3938 w3979 w4020 w4061 w4102 w4143 w4184 w4225 w4266 w4307 w4348 w4389 w4430 w4471 w4512 w4553 w4594 w4635 w4676 w4717 w4758 w4799 w4840 w4881 w4922 w4963 w5004 w5045 w5086 w5127 w5168 w5209 w5250 w5291 w5332 w5373 w5414 w5455 w5496 w5537 w5578 w5619 w5660 w5694 w5742 w5799 w5856 w5913 w5970 w6027 w6084 w6141 w6198 w6255 w6312 w6369 w6426 w6483 w6540 w6597 w6654 w6711 w6768 w6825 w6882 w6939 w6996 w7053 w7110 w7167 w7224 w7281 w7338 w7395 w7452 w7509 w7566 w7623 w7680 w7737 w7794 w7851 w7908 w7965 w8022 w8079 w8136 w8193 w8250 w8307 w8364 w8421 w8478 w8535 w8592 w8649 w8706 w8763 w8820 w8877 w8936 w8995 w9054 w9113]
      tunnel: [w281 w1313 w1326 w1339 w1359 w1420 w1452 w1500 w1544 w1556 w1568 w1586 w1607 w1637 w1656 w1726 w1749 w1772 w1795 w1811 w1846 w1865 w1884 w1904 w1937 w1973 w1992 w2019 w2055 w2079 w2098 w2133 w2153 w2177 w2220 w2245 w2284 w2334 w2369 w2426 w2485 w2556 w2627 w2698 w2769 w2840 w2911 w2982 w3016 w3124 w3201 w3241 w3282 w3323 w3364 w3405 w3446 w3487 w3528 w3569 w3610 w3651 w3692 w3733 w3774 w3815 w3856 w3897 w3938 w3979 w4020 w4061 w4102 w4143 w4184 w4225 w4266 w4307 w4348 w4389 w4430 w4471 w4512 w4553 w4594 w4635 w4676 w4717 w4758 w4799 w4840 w4881 w4922 w4963 w5004 w5045 w5086 w5127 w5168 w5209 w5250 w5291 w5332 w5373 w5414 w5455 w5496 w5537 w5578 w5619 w5660 w5694 w5742 w5799 w5856 w5913 w5970 w6027 w6084 w6141 w6198 w6255 w6312 w6369 w6426 w6483 w6540 w6597 w6654 w6711 w6768 w6825 w6882 w6939 w6996 w7053 w7110 w7167 w7224 w7281 w7338 w7395 w7452 w7509 w7566 w7623 w7680 w7737 w7794 w7851 w7908 w7965 w8022 w8079 w8136 w8193 w8250 w8307 w8364 w8421 w8478 w8535 w8592 w8649 w8706 w8763 w8820 w8877 w8936 w8995 w9054 w9113] -> w244
      tunnel: w243 -> [w280 w1312 w1325 w1338 w1358 w1419 w1451 w1499 w1543 w1555 w1567 w1585 w1606 w1636 w1655 w1725 w1745 w1769 w1791 w1812 w1845 w1862 w1883 w1903 w1936 w1972 w1991 w2018 w2054 w2078 w2097 w2132 w2152 w2176 w2219 w2244 w2283 w2333 w2368 w2425 w2484 w2555 w2626 w2697 w2768 w2839 w2910 w2981 w3053 w3123 w3200 w3240 w3281 w3322 w3363 w3404 w3445 w3486 w3527 w3568 w3609 w3650 w3691 w3732 w3773 w3814 w3855 w3896 w3937 w3978 w4019 w4060 w4101 w4142 w4183 w4224 w4265 w4306 w4347 w4388 w4429 w4470 w4511 w4552 w4593 w4634 w4675 w4716 w4757 w4798 w4839 w4880 w4921 w4962 w5003 w5044 w5085 w5126 w5167 w5208 w5249 w5290 w5331 w5372 w5413 w5454 w5495 w5536 w5577 w5618 w5659 w5693 w5741 w5798 w5855 w5912 w5969 w6026 w6083 w6140 w6197 w6254 w6311 w6368 w6425 w6482 w6539 w6596 w6653 w6710 w6767 w6824 w6881 w6938 w6995 w7052 w7109 w7166 w7223 w7280 w7337 w7394 w7451 w7508 w7565 w7622 w7679 w7736 w7793 w7850 w7907 w7964 w8021 w8078 w8135 w8192 w8249 w8306 w8363 w8420 w8477 w8534 w8591 w8648 w8705 w8762 w8819 w8876 w8935 w8994 w9053 w9112]
      tunnel: [w280 w1312 w1325 w1338 w1358 w1419 w1451 w1499 w1543 w1555 w1567 w1585 w1606 w1636 w1653 w1725 w1745 w1769 w1791 w1812 w1845 w1862 w1883 w1903 w1936 w1972 w1991 w2018 w2054 w2078 w2097 w2132 w2152 w2176 w2219 w2244 w2283 w2333 w2368 w2425 w2484 w2555 w2626 w2697 w2768 w2839 w2910 w2981 w3053 w3123 w3200 w3240 w3281 w3322 w3363 w3404 w3445 w3486 w3527 w3568 w3609 w3650 w3691 w3732 w3773 w3814 w3855 w3896 w3937 w3978 w4019 w4060 w4101 w4142 w4183 w4224 w4265 w4306 w4347 w4388 w4429 w4470 w4511 w4552 w4593 w4634 w4675 w4716 w4757 w4798 w4839 w4880 w4921 w4962 w5003 w5044 w5085 w5126 w5167 w5208 w5249 w5290 w5331 w5372 w5413 w5454 w5495 w5536 w5577 w5618 w5659 w5693 w5741 w5798 w5855 w5912 w5969 w6026 w6083 w6140 w6197 w6254 w6311 w6368 w6425 w6482 w6539 w6596 w6653 w6710 w6767 w6824 w6881 w6938 w6995 w7052 w7109 w7166 w7223 w7280 w7337 w7394 w7451 w7508 w7565 w7622 w7679 w7736 w7793 w7850 w7907 w7964 w8021 w8078 w8135 w8192 w8249 w8306 w8363 w8420 w8477 w8534 w8591 w8648 w8705 w8762 w8819 w8876 w8935 w8994 w9053 w9112] -> w242
      tunnel: w241 -> [w264 _ _ _ w1347 _ _ _ _ _ w1560 _ _ _ _ _ _ _ _ _ _ _ _ _ _ w1971 _ _ _ w2075 _ _ w2151 w2175 w2218 w2233 w2282 w2332 _ _ _ _ _ _ _ _ _ _ _ _ _ _ _ _ _ _ _ _ _ _ _ _ _ _ _ _ _ _ _ _ _ _ _ _ _ _ _ _ _ _ _ _ _ _ _ _ _ _ _ _ _ _ _ _ _ _ _ _ _ _ _ _ _ _ _ _ _ _ _ _ _ _ _ _ _ _ _ _ _ _ _ _ _ _ _ _ _ _ _ _ _ _ _ _ _ _ _ _ _ _ _ _ _ _ _ _ _ _ _ _ _ _ _ _ _ _ _ _ _ _ _ _ _ _ _ _ _ _ _ _ _ _]
      tunnel: w231 -> [w277 _ w1321 w1337 _ _ w1431 _ _ _ _ _ w1603 _ w1643 w1712 _ _ _ _ _ _ _ _ w1916 _ _ _ _ _ _ _ _ _ _ _ _ _ _ w2415 w2451 w2521 w2592 w2662 w2734 w2804 w2877 w2948 w3019 w3092 w3171 w3235 w3276 w3317 w3358 w3399 w3440 w3481 w3522 w3563 w3604 w3645 w3686 w3727 w3768 w3809 w3850 w3891 w3932 w3973 w4014 w4055 w4096 w4137 w4178 w4219 w4260 w4301 w4342 w4383 w4424 w4465 w4506 w4547 w4588 w4629 w4670 w4711 w4752 w4793 w4834 w4875 w4916 w4957 w4998 w5039 w5080 w5121 w5162 w5203 w5244 w5285 w5326 w5367 w5408 w5449 w5490 w5531 w5572 w5613 w5654 _ w5708 w5765 w5822 w5879 w5936 w5993 w6050 w6107 w6164 w6221 w6278 w6335 w6392 w6449 w6507 w6564 w6621 w6678 w6735 w6792 w6849 w6906 w6963 w7020 w7077 w7134 w7191 w7248 w7305 w7362 w7419 w7476 w7533 w7590 w7647 w7704 w7761 w7819 w7875 w7932 w7989 w8046 w8103 w8160 w8217 w8274 w8333 w8388 w8445 w8502 w8559 w8616 w8674 w8730 w8787 w8844 w8904 w8963 w9022 w9081]
      tunnel: [w276 w1311 w1324 w1335 w1351 w1412 w1450 w1498 w1542 w1554 w1566 w1579 w1605 w1635 w1652 w1724 w1739 w1762 w1785 w1810 w1844 w1863 w1881 w1900 w1934 w1964 w1990 w2017 w2053 w2073 w2096 w2130 w2149 w2173 w2216 w2243 w2280 w2330 w2367 w2424 w2465 w2537 w2607 w2678 w2749 w2820 w2891 w2962 w3034 w3107 w3184 w3239 w3280 w3321 w3362 w3403 w3444 w3485 w3526 w3567 w3608 w3649 w3690 w3731 w3772 w3813 w3854 w3895 w3936 w3977 w4018 w4059 w4100 w4141 w4182 w4223 w4264 w4305 w4346 w4387 w4428 w4469 w4510 w4551 w4592 w4633 w4674 w4715 w4756 w4797 w4838 w4879 w4920 w4961 w5002 w5043 w5084 w5125 w5166 w5207 w5248 w5289 w5330 w5371 w5412 w5453 w5494 w5535 w5576 w5617 w5658 w5692 w5740 w5797 w5854 w5911 w5968 w6025 w6082 w6139 w6196 w6253 w6310 w6367 w6424 w6481 w6538 w6595 w6652 w6709 w6766 w6823 w6880 w6937 w6994 w7051 w7108 w7165 w7222 w7279 w7336 w7393 w7450 w7507 w7564 w7621 w7678 w7735 w7792 w7849 w7906 w7963 w8020 w8077 w8134 w8191 w8248 w8305 w8362 w8419 w8476 w8533 w8590 w8647 w8704 w8761 w8818 w8875 w8934 w8993 w9052 w9111] -> w240
      tunnel: w239 -> [w275 w1311 w1324 w1335 w1351 w1412 w1450 w1498 w1542 w1554 w1566 w1579 w1605 w1635 w1652 w1724 w1739 w1762 w1785 w1810 w1844 w1863 w1881 w1900 w1934 w1964 w1990 w2017 w2053 w2073 w2096 w2130 w2149 w2173 w2216 w2243 w2280 w2330 w2367 w2424 w2465 w2537 w2607 w2678 w2749 w2820 w2891 w2962 w3034 w3107 w3184 w3239 w3280 w3321 w3362 w3403 w3444 w3485 w3526 w3567 w3608 w3649 w3690 w3731 w3772 w3813 w3854 w3895 w3936 w3977 w4018 w4059 w4100 w4141 w4182 w4223 w4264 w4305 w4346 w4387 w4428 w4469 w4510 w4551 w4592 w4633 w4674 w4715 w4756 w4797 w4838 w4879 w4920 w4961 w5002 w5043 w5084 w5125 w5166 w5207 w5248 w5289 w5330 w5371 w5412 w5453 w5494 w5535 w5576 w5617 w5658 w5692 w5740 w5797 w5854 w5911 w5968 w6025 w6082 w6139 w6196 w6253 w6310 w6367 w6424 w6481 w6538 w6595 w6652 w6709 w6766 w6823 w6880 w6937 w6994 w7051 w7108 w7165 w7222 w7279 w7336 w7393 w7450 w7507 w7564 w7621 w7678 w7735 w7792 w7849 w7906 w7963 w8020 w8077 w8134 w8191 w8248 w8305 w8362 w8419 w8476 w8533 w8590 w8647 w8704 w8761 w8818 w8875 w8934 w8993 w9052 w9111]
      tunnel: w237 -> [w274 _ _ _ w1353 w1407 _ w1486 _ _ _ _ _ _ _ _ _ _ _ _ _ _ _ _ _ _ _ _ _ _ _ w2124 _ _ _ _ _ _ _ w2414 _ _ _ _ _ _ _ _ _ _ _ _ _ _ _ _ _ _ _ _ _ _ _ _ _ _ _ _ _ _ _ _ _ _ _ _ _ _ _ _ _ _ _ _ _ _ _ _ _ _ _ _ _ _ _ _ _ _ _ _ _ _ _ _ _ _ _ _ _ _ _ _ w5697 w5754 w5811 w5869 w5925 w5983 w6040 w6097 w6154 w6211 w6268 w6325 w6381 w6438 w6495 w6552 w6609 w6666 w6723 w6780 w6838 w6894 w6952 w7009 w7065 w7123 w7179 w7237 w7293 w7351 w7408 w7465 w7521 w7578 w7636 w7693 w7750 w7807 w7864 w7921 w7978 w8035 w8092 w8150 w8206 w8262 w8320 w8378 w8435 w8492 w8548 w8605 w8662 w8719 w8776 w8833 w8894 w8953 w9012 w9071]
